vi "GetSignalParams.vi"(8 "error in (no error)":errorcluster, 11 "StandardFunction in":refnum<class "StandardFunction.lvclass">) -> (0 "error out":errorcluster, 2 "Params":variant, 3 "StandardFunction out":refnum<class "StandardFunction.lvclass">)   [LabVIEW 2018, in "Functions.lvlib" / "StandardFunction.lvclass"]
uses:
  StandardFunction.lvclass
  StandardFunction.lvclass/StandardFunction.ctl
  Accessors/Read StandardWfrms.vi
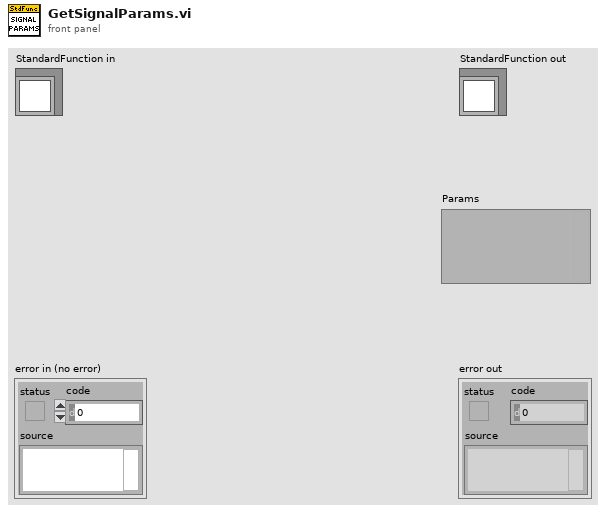
[diagram p1: front panel]
types:
  T1 = typedef "Functions.lvlib/StandardFunction.lvclass/StdWfrms.ctl" = cluster{"Count":u16, "StandardWfrm":T2[]}
  T2 = typedef "Functions.lvlib/StandardFunction.lvclass/StdWfrm.ctl" = cluster{"Amplitude":dbl, "DcOffset":dbl, "DutyCycle":dbl, "Frequency":dbl, "Phase":dbl, "Waveform":enum16{"Sine", "Square", "Triangle", "Ramp Up", "Ramp Down", "DC"}, "Handle":string}
  T3 = enum16{"Sine", "Square", "Triangle", "Ramp Up", "Ramp Down", "DC"}
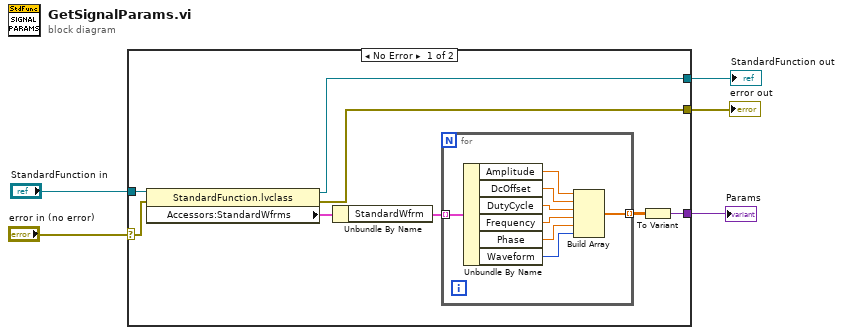
[diagram p0: block diagram]
diagram:
  n1 = case shown="No Error" "error in (no error)" {
    selector: "error in (no error)" -> [w12 w22]
    tunnel: "StandardFunction in" -> [w13 w23]
    tunnel: [w8 _] -> w3
    tunnel: [w7 w23] -> w2
    tunnel: [w6 w22] -> w1
    frame No Error {
      n2 = property class="StandardFunction.lvclass"(reference=w13, error in=w12) -> (reference out=w7:refnum<class "StandardFunction.lvclass">, error out=w6:errorcluster, "Accessors:StandardWfrms"=w11:T1)
      n3 = Unbundle By Name(w11) -> ("StandardWfrm"=w10:T2[])
      n4 = for {
        tunnel: w10 -> [w21] mode=indexing
        tunnel: [w14] -> w9 mode=indexing
        n5 = Unbundle By Name(w21) -> ("Amplitude"=w17:dbl, "DcOffset"=w18:dbl, "DutyCycle"=w20:dbl, "Frequency"=w19:dbl, "Phase"=w16:dbl, "Waveform"=w15:T3)
        n6 = Build Array(w17, w18, w20, w19, w16, w15) -> (w14:dbl[])
      }
      n7 = To Variant(anything=w9) -> (Variant=w8:variant)
    }
    frame Error {
    }
  }
  "error out" <- w1
  "StandardFunction out" <- w2
  "Params" <- w3
